vi "PC Vg Sweep.vi"() -> ()   [LabVIEW 2009]
uses:
  <vilib>/DAQmx/create/channels.llb/DAQmx Create Channel (AO-Voltage-Basic).vi
  <vilib>/DAQmx/create/channels.llb/DAQmx Create Channel (AI-Voltage-Basic).vi
  <vilib>/DAQmx/configure/timing.llb/DAQmx Timing (Sample Clock).vi
  <vilib>/DAQmx/write.llb/DAQmx Write (Analog DBL 1Chan 1Samp).vi
  <vilib>/DAQmx/read.llb/DAQmx Read (Analog 1D DBL 1Chan NSamp).vi
  <vilib>/Utility/file.llb/Write To Spreadsheet File (DBL).vi
  <vilib>/Analysis/NI_AALBase.lvlib
panel:
  in  "Stop":bool
  out "Vg":dbl(graph)
  out "Vsd":dbl(graph)
  out "Writing Vsd":bool
  out "Start Vsd Ramp":bool=TRUE
  in  "Measured Current":tag
  in  "Save Spectral?":bool
  in  "Save Map?":bool
  out "Mono Outputs":T1
  in  "Select Grating Blaze":string(combo)
  in  "Force\nInitialization (Def: F)":bool
  in  "Mono ID":string(combo)
  in  "Current Map":path
  in  "Spectral Response":path
  out "Current vs Wavelength":cluster{dbl[], dbl[]}(graph)
  out "Current vs Gate Voltage":cluster{dbl[], dbl[]}(graph)
  out "Out of Range":bool
  out "Vsd Ramp Position":cluster{"Vsd On":dbl, "Vsd On Vg Dir":bool}
  out "Recording":bool=TRUE
  out "Direction":bool=TRUE
  in  "Start Scan":bool
  out "Vsd Value (V)":dbl format="%0.2f"
  out "Vg Value (V)":dbl format="%0.2f"
  in  "Scan Values":T2={"Min Vg (V)"=0.0, "Max Vg (V)"=10.0, "Vm Start (V)"=5.0, "Vm Stop (V)"=9.0, "Steps/Sec"=100.0, "Vm Rate (Hz)"=100.0, "Wavelength Start (nm)"=450.0, "Wavelength Stop (nm)"=850.0, "Wavelength Step (nm)"=2.0, "Vsd (V)"=0.1, "Vg Step Size"=0.01, "Vsd Ramp Time (secs)"=0.1} {"Vsd Ramp Time (secs)" min=-10.0 max=10.0; "Vg Step Size" min=0.0 max=0.5; "Vsd (V)" min=-10.0 max=10.0; "Wavelength Step (nm)" min=0.0 max=500.0; "Wavelength Stop (nm)" min=16.0 max=2500.0; "Wavelength Start (nm)" min=15.0 max=2499.0; "Steps/Sec" min=1.0 max=1000.0; "Vm Stop (V)" min=-10.0 max=10.0; "Vm Start (V)" min=-10.0 max=10.0; "Max Vg (V)" min=-9.9 max=10.0; "Min Vg (V)" min=-10.0 max=9.9}
  in  "Start Mono":bool
  in  "Gate Voltage":tag
  in  "Source Drain Bias":tag
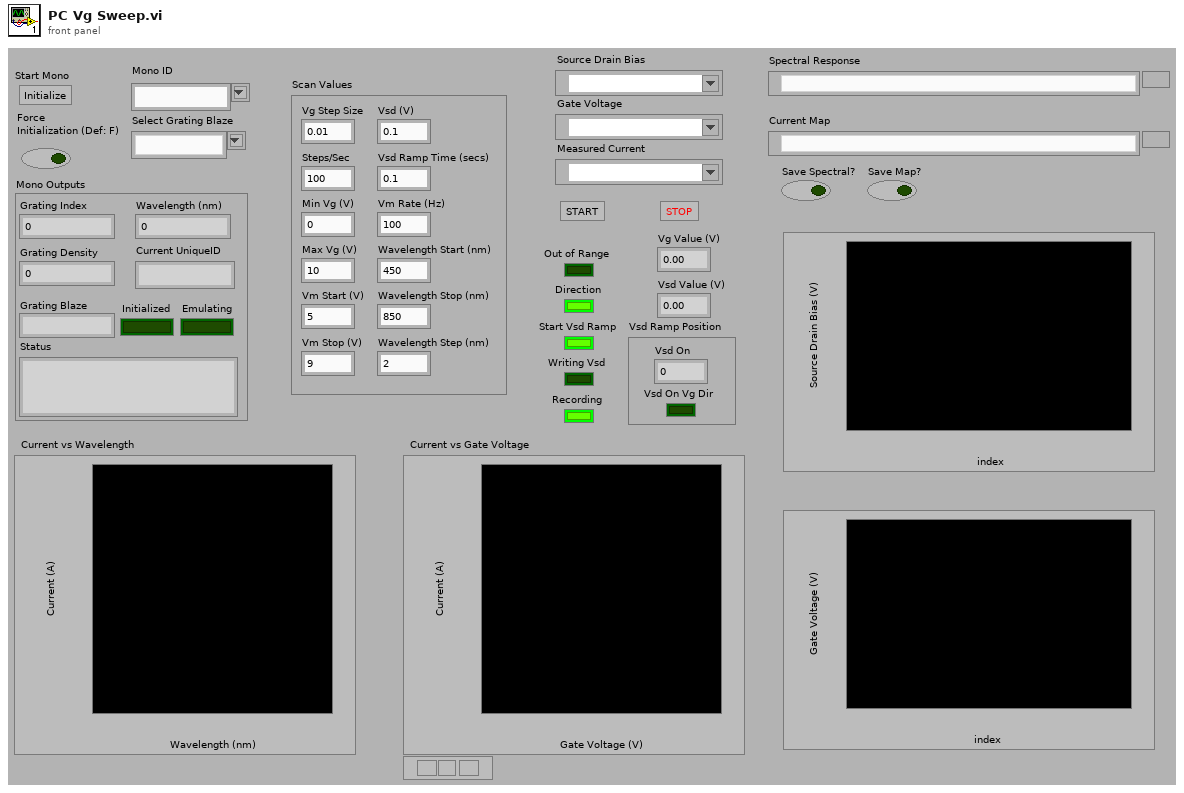
[diagram p1: front panel]
types:
  T1 = cluster{"Current UniqueID":string, "Current Blaze":string, "Grating Density":dbl, "Grating Index":i32, "Wavelength (nm)":dbl, "Emulating":bool, "Initialized":bool, "Status":string, "Refnum out":refnum<k7>}
  T2 = cluster{"Min Vg (V)":dbl, "Max Vg (V)":dbl, "Vm Start (V)":dbl, "Vm Stop (V)":dbl, "Steps/Sec":dbl, "Vm Rate (Hz)":dbl, "Wavelength Start (nm)":dbl, "Wavelength Stop (nm)":dbl, "Wavelength Step (nm)":dbl, "Vsd (V)":dbl, "Vg Step Size":dbl, "Vsd Ramp Time (secs)":dbl}
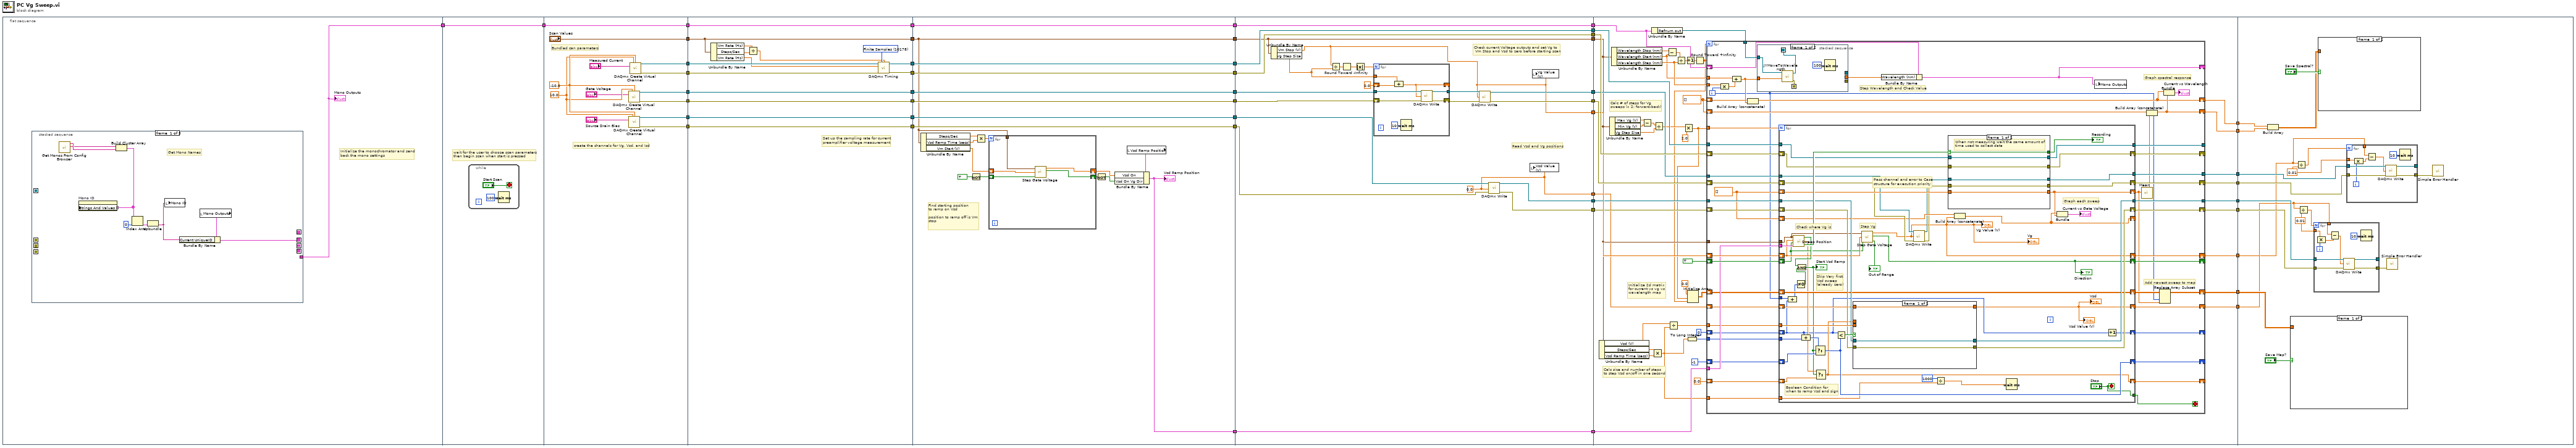
[diagram p0: block diagram]
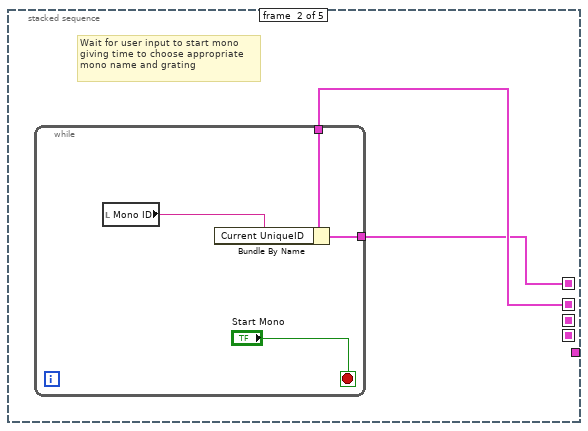
[diagram p2: hidden frame]
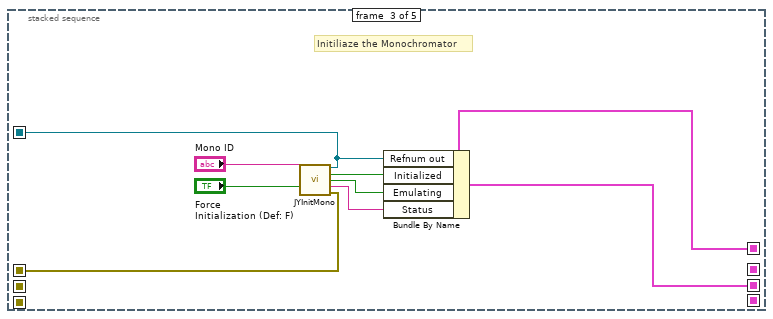
[diagram p3: hidden frame]
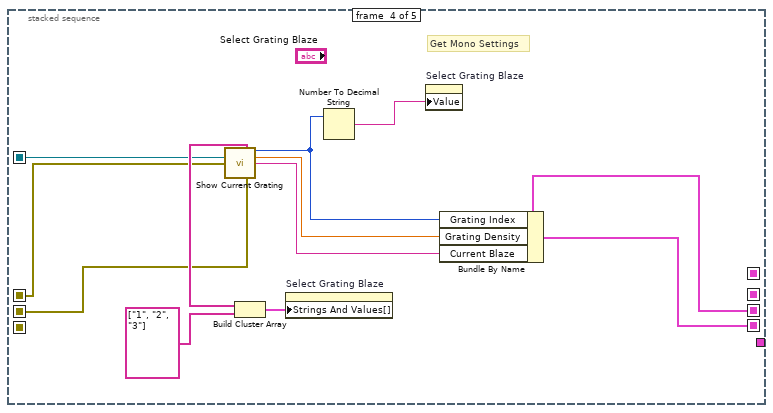
[diagram p4: hidden frame]
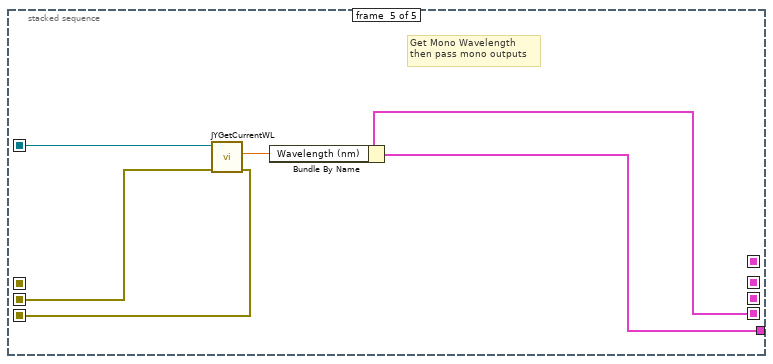
[diagram p5: hidden frame]
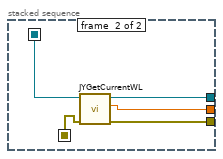
[diagram p6: hidden frame]
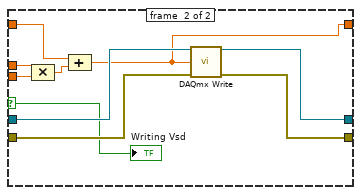
[diagram p7: hidden frame]
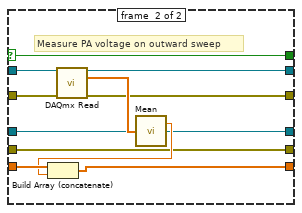
[diagram p8: hidden frame]
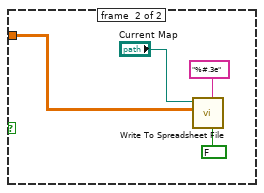
[diagram p9: hidden frame]
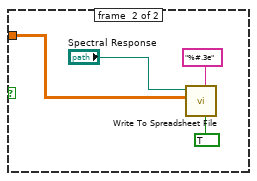
[diagram p10: hidden frame]
diagram:
  n1 = flat-sequence {
    tunnel: [w48] -> w2
    tunnel: w2 -> [w90]
    tunnel: [w90] -> w1
    tunnel: w1 -> [w101]
    tunnel: [w101] -> w47
    tunnel: ["Scan Values"] -> w46
    tunnel: [w99] -> w45
    tunnel: [w98] -> w44
    tunnel: [w97] -> w43
    tunnel: [w96] -> w42
    tunnel: [w95] -> w41
    tunnel: [w94] -> w40
    tunnel: [w120] -> w29
    tunnel: [w110] -> w27
    tunnel: [w119] -> w25
    tunnel: [w118] -> w23
    tunnel: [w117] -> w21
    tunnel: [w116] -> w19
    tunnel: [w114] -> w17
    tunnel: [w115] -> w15
    tunnel: w40 -> [w113]
    tunnel: w41 -> [w112]
    tunnel: w42 -> [w116]
    tunnel: w43 -> [w117]
    tunnel: w44 -> [w118]
    tunnel: w45 -> [w119]
    tunnel: w46 -> [w110]
    tunnel: w47 -> [w120]
    tunnel: w29 -> [w139]
    tunnel: [w139] -> w28
    tunnel: w27 -> [w132]
    tunnel: [w132] -> w26
    tunnel: w25 -> [w138]
    tunnel: [w138] -> w24
    tunnel: w23 -> [w137]
    tunnel: [w137] -> w22
    tunnel: w21 -> [w136]
    tunnel: [w136] -> w20
    tunnel: w19 -> [w135]
    tunnel: [w135] -> w18
    tunnel: w17 -> [w134]
    tunnel: [w134] -> w16
    tunnel: w15 -> [w133]
    tunnel: [w133] -> w14
    tunnel: [w125] -> w13
    tunnel: w28 -> [w164]
    tunnel: w26 -> [w158]
    tunnel: w24 -> [w149]
    tunnel: w22 -> [w153]
    tunnel: w20 -> [w148]
    tunnel: w18 -> [w152]
    tunnel: w16 -> [w162]
    tunnel: w14 -> [w163]
    tunnel: [w164] -> w39
    tunnel: [w145] -> w38
    tunnel: [w146] -> w37
    tunnel: [w155] -> w36
    tunnel: [w154] -> w35
    tunnel: [w163] -> w34
    tunnel: [w162] -> w33
    tunnel: [w150] -> w32
    tunnel: [w147] -> w31
    tunnel: [w158] -> w30
    tunnel: w13 -> [w156]
    tunnel: [w156] -> w12
    tunnel: w33 -> [w216]
    tunnel: w34 -> [w215]
    tunnel: w39 -> [w217]
    tunnel: w32 -> [w208]
    tunnel: w36 -> [w209]
    tunnel: w35 -> [w210]
    tunnel: w31 -> [w197]
    tunnel: w38 -> [w206]
    tunnel: w37 -> [w205]
    tunnel: w30 -> [w199]
    tunnel: w12 -> [w202]
    tunnel: [w189] -> w11
    tunnel: [w188] -> w10
    tunnel: [w187] -> w9
    tunnel: [w186] -> w8
    tunnel: [w185] -> w7
    tunnel: [w184] -> w6
    tunnel: [w183] -> w5
    tunnel: [w182] -> w4
    tunnel: [w181] -> w3
    tunnel: w11 -> [w380]
    tunnel: w10 -> [w379]
    tunnel: w9 -> [w377]
    tunnel: w8 -> [w370]
    tunnel: w7 -> [w369]
    tunnel: w6 -> [w368]
    tunnel: w5 -> [w367]
    tunnel: w4 -> [w366]
    tunnel: w3 -> [w365]
    frame #0 {
      # "Initialize the monochromator and send\nback the mono settings"
      n2 = stacked-sequence {
        seq-local: [_ _ w70 _ _] -> [_ _ _ w79 _]
        seq-local: [_ _ w69 _ _] -> [_ _ _ w78 w89]
        seq-local: [_ _ _ w77 _] -> [_ _ _ _ w88]
        seq-local: [_ _ _ _ w87] -> [_ _ _ _ _]
        seq-local: [w49 _ _ _ _] -> [_ w58 _ _ _]
        seq-local: [_ _ w64 _ _] -> [_ _ _ w76 _]
        seq-local: [_ _ _ w72 _] -> [_ _ _ _ w86]
        seq-local: [_ w57 _ _ _] -> [_ _ w63 _ _]
        tunnel: [_ _ _ _ w84] -> w48
        frame #0 {
          # "Get Mono Names"
          n3 = call "Get Monos From Config Browser.vi"() -> ("UniqueIDs"=w53:string[], "Mono ID"=w52:string[])  [unwired: 3 in, 1 out]
          n4 = Build Cluster Array(w52, w53) -> (w55:cluster{"String":string, "String":string}[])
          n5 = property on="Mono ID" class="CmbBox"("Strings And Values []"=w55) -> ()  [unwired: 2 in, 2 out]
          n6 = Index Array(array=w55, index=0) -> (element=w54:cluster{"String":string, "String":string})
          n7 = Unbundle(w54) -> ("String"=w50:string)  [unwired: 1 out]
          n8 = local write "Mono ID"(w50) -> ()
          n9 = local read "Mono Outputs"() -> (w51:T1)
          n10 = Bundle By Name(cluster=w51, "Current UniqueID"=w50) -> (w49:T1)
        }
        frame #1 {
          # "Wait for user input to start mono\ngiving time to choose appropriate\nmono name and grating"
          n11 = while {
            tunnel: w58 -> [w61]
            tunnel: [w59] -> w57
            stop <- "Start Mono" stop-if-true
            n12 = local read "Mono ID"() -> (w60:string)
            n13 = Bundle By Name(cluster=w61, "Current UniqueID"=w60) -> (w59:T1)
          }
        }
        frame #2 {
          # "Initiliaze the Monochromator"
          n14 = call "JYInitMono.vi"("Unique ID"="Mono ID", "Force Init"="Force\nInitialization (Def: F)") -> ("Mono RefNum out"=w69:refnum<k7>, "Initialized"=w68:bool, "Emulating"=w67:bool, "Status"=w66:string, "error out"=w70:errorcluster)  [unwired: 9 in]
          n15 = Bundle By Name(cluster=w63, "Refnum out"=w69, "Initialized"=w68, "Emulating"=w67, "Status"=w66) -> (w64:T1)
        }
        frame #3 {
          # "Get Mono Settings"
          n16 = call "Show Current Grating.vi"("Refnum in"=w78, "error in (no error)"=w79) -> ("Blazes"=w82:string[], "Grating Index"=w75:i32, "Current Grating"=w74:dbl, "Current Blaze"=w73:string, "error out"=w77:errorcluster)  [unwired: 5 in, 4 out]
          n17 = Build Cluster Array(w82, string[] ["1", "2", "3"]) -> (w80:cluster{"String":string, string}[])
          n18 = property on="Select Grating Blaze" class="CmbBox"("Strings And Values[]"=w80) -> ()  [unwired: 2 in, 2 out]
          n19 = Number To Decimal String(number=w75) -> (decimal integer string=w83:string)  [unwired: 1 in]
          n20 = property on="Select Grating Blaze" class="CmbBox"("Value"=w83) -> ()  [unwired: 2 in, 2 out]
          n21 = Bundle By Name(cluster=w76, "Grating Index"=w75, "Grating Density"=w74, "Current Blaze"=w73) -> (w72:T1)
        }
        frame #4 {
          # "Get Mono Wavelength\nthen pass mono outputs"
          n22 = call "JYGetCurrentWL.vi"("error in (no error)"=w88, "JYMONOLib.IJYMonoReqd"=w89) -> ("error out"=w87:errorcluster, "Current WL"=w85:dbl)  [unwired: 6 in, 2 out]
          n23 = Bundle By Name(cluster=w86, "Wavelength (nm)"=w85) -> (w84:T1)
        }
      }
      "Mono Outputs" <- w48
    }
    frame #1 {
      # "wait for the user to choose scan parameters\nthen begin scan when start is pressed"
      n24 = while {
        stop <- "Start Scan" stop-if-true
        n25 = Wait (ms)(milliseconds to wait=u32 100) -> ()  [unwired: 1 out]
      }
    }
    frame #2 {
      w105 = -10.0 ("maximum value")
      w104 = 10.0 ("maximum value")
      # "create the channels for Vg, Vsd, and Isd"
      # "Bundled can parameters"
      n26 = call-poly <vilib>:"DAQmx Create Virtual Channel.vi"("maximum value"=w104, "minimum value"=w105, "physical channels"="Gate Voltage") -> ("task out"=w98:refnum<k21>, "error out"=w96:errorcluster)  [unwired: 11 in]
      n27 = call-poly <vilib>:"DAQmx Create Virtual Channel.vi"("maximum value"=w104, "minimum value"=w105, "physical channels"="Source Drain Bias") -> ("task out"=w99:refnum<k21>, "error out"=w97:errorcluster)  [unwired: 11 in]
      n28 = call-poly <vilib>:"DAQmx Create Virtual Channel.vi"("maximum value"=w104, "minimum value"=w105, "physical channels"="Measured Current") -> ("task out"=w94:refnum<k21>, "error out"=w95:errorcluster)  [unwired: 11 in]
    }
    frame #3 {
      w111 = 10178 items=["Finite Samples"=10178, "Continuous Samples"=10123, "Hardware Timed Single Point"=12522] ("sample mode")
      # "Set up the sampling rate for current\npreamplifier voltage measurement"
      n29 = Unbundle By Name(w110) -> ("Vm Rate (Hz)"=w108:dbl, "Steps/Sec"=w109:dbl, "Vm Rate (Hz)"=w106:dbl)
      n30 = Divide(x=w108, y=w109) -> (x/y=w107:dbl)
      n31 = call-poly <vilib>:"DAQmx Timing.vi"("task/channels in"=w113, "sample mode"=w111, "samples per channel"=w107, "rate"=w106, "error in"=w112) -> ("task out"=w115:refnum<k21>, "error out"=w114:errorcluster)  [unwired: 9 in]
    }
    frame #4 {
      # "Find starting position\nto ramp on Vsd\n\nposition to ramp off is Vm\nstop"
      n32 = Unbundle By Name(w132) -> ("Steps/Sec"=w122:dbl, "Vsd Ramp Time (secs)"=w123:dbl, "Vm Start (V)"=w124:dbl)
      n33 = Not(x=TRUE ("Direction")) -> (.not. x?=w131:bool)
      n34 = Multiply(x=w122, y=w123) -> (x*y=w121:dbl)
      n35 = for {
        N: w121 -> [_]
        tunnel: w132 -> [w140]
        shift-right: [w143] -> w126
        shift-left: w124 -> [w144]
        shift-right: [w141] -> w129
        shift-left: w131 -> [w142]
        n36 = call "Step Gate Voltage.vi"("Scan Values"=w140, "Vg Value (V)"=w144, "Direction"=w142) -> ("New Vg Value (V)"=w143:dbl, "New Direction"=w141:bool)  [unwired: 2 out]
      }
      n37 = Not(x=w129) -> (.not. x?=w127:bool)
      n38 = local read "Vsd Ramp Position"() -> (w128:cluster{"Vsd On":dbl, "Vsd On Vg Dir":bool})
      n39 = Bundle By Name(cluster=w128, "Vsd On"=w126, "Vsd On Vg Dir"=w127) -> (w125:cluster{"Vsd On":dbl, "Vsd On Vg Dir":bool})
      "Vsd Ramp Position" <- w125
    }
    frame #5 {
      w147 = 0.0 ("data")
      # "Read Vsd and Vg positions"
      # "Check current Voltage outputs and set Vg to\n Vm Stop and Vsd to zero before starting scan"
      n40 = Unbundle By Name(w158) -> ("Vm Stop (V)"=w150:dbl, "Vg Step Size"=w157:dbl)
      n41 = Divide(x=w150, y=w157) -> (x/y=w161:dbl)
      n42 = Round Toward -Infinity(1:w161) -> (0:w160:dbl)
      n43 = Absolute Value(x=w160) -> (abs(x)=w159:dbl)
      n44 = for {
        N: w159 -> [_]
        tunnel: w153 -> [w174]
        tunnel: w157 -> [w167]
        tunnel: [w171] -> w166
        shift-right: [w170] -> w165
        shift-left: w152 -> [w173]
        shift-right: [w168] -> _
        shift-left: 0.0 -> [w169]
        n45 = Compound Arithmetic op=ADD(w167, w169) -> (w168:dbl)
        n46 = Wait (ms)(milliseconds to wait=u32 10) -> ()  [unwired: 1 out]
        n47 = call-poly <vilib>:"DAQmx Write.vi"("task/channels in"=w174, "data"=w168, "error in"=w173) -> ("task out"=w171:refnum<k21>, "error out"=w170:errorcluster)  [unwired: 10 in, 1 out]
      }
      n48 = call-poly <vilib>:"DAQmx Write.vi"("task/channels in"=w166, "data"=w150, "error in"=w165) -> ("task out"=w155:refnum<k21>, "error out"=w154:errorcluster)  [unwired: 10 in, 1 out]
      n49 = call-poly <vilib>:"DAQmx Write.vi"("task/channels in"=w149, "data"=w147, "error in"=w148) -> ("task out"=w145:refnum<k21>, "error out"=w146:errorcluster)  [unwired: 10 in, 1 out]
      n50 = local write "Vsd Value (V)"(w147) -> ()
      n51 = local write "Vg Value (V)"(w150) -> ()
    }
    frame #6 {
      w190 = dbl[] []
      # "Initialize 2d matrix\nfor current vs vg vs \nwavelength map"
      # "Calc # of steps for Vg\nsweeps (x 2: forward-back)"
      # "Calc size and number of steps\nto step Vsd on/off in one second"
      n52 = Unbundle By Name(w199) -> ("Vsd (V)"=w196:dbl, "Steps/Sec"=w177:dbl, "Vsd Ramp Time (secs)"=w176:dbl)
      n53 = Unbundle By Name(w199) -> ("Max Vg (V)"=w211:dbl, "Min Vg (V)"=w212:dbl, "Vg Step Size"=w213:dbl)
      n54 = Unbundle By Name(w199) -> ("Wavelength Stop (nm)"=w222:dbl, "Wavelength Start (nm)"=w219:dbl, "Wavelength Step (nm)"=w220:dbl)
      n55 = Subtract(x=w211, y=w212) -> (x-y=w214:dbl)
      n56 = Unbundle By Name(w217) -> ("Refnum out"=w218:refnum<k7>)
      n57 = Multiply(x=w177, y=w176) -> (x*y=w175:dbl)
      n58 = Divide(x=w214, y=w213) -> (x/y=w204:dbl)
      n59 = Subtract(x=w222, y=w219) -> (x-y=w221:dbl)
      n60 = Divide(x=w196, y=w175) -> (x/y=w195:dbl)
      n61 = Divide(x=w221, y=w220) -> (x/y=w201:dbl)
      n62 = Multiply(x=w204, y=2.0) -> (x*y=w192:dbl)
      n63 = Increment(x=w201) -> (x+1=w200:dbl)
      n64 = To Long Integer(number=w175) -> (32bit integer=w198:i32)
      n65 = Round Toward +Infinity(x=w200) -> (ceil(x): smallest int >= x=w193:dbl)
      n66 = Initialize Array(0.0, w192, w193) -> (w191:dbl[][])
      n67 = for {
        N: w193 -> [_]
        tunnel: w220 -> [w273]
        tunnel: w219 -> [w271]
        tunnel: w218 -> [w270]
        shift-right: [w233] -> _
        shift-left: w217 -> [w269]
        shift-right: [w238] -> w189
        shift-left: w190 -> [w244]
        shift-right: [w247] -> w183
        shift-left: w205 -> [w259]
        shift-right: [w246] -> w185
        shift-left: w210 -> [w266]
        tunnel: w206 -> [w260]
        tunnel: w209 -> [w267]
        tunnel: w215 -> [w256]
        shift-right: [w245] -> _
        shift-left: w216 -> [w255]
        tunnel: w198 -> [w254]
        tunnel: w192 -> [w265]
        shift-right: [w261] -> w181
        shift-left: w208 -> [w263]
        shift-right: [w262] -> _
        shift-left: TRUE -> [w264]
        tunnel: w202 -> [w258]
        tunnel: w199 -> [w257]
        shift-right: [w252] -> w182
        shift-left: w197 -> [w253]
        tunnel: w195 -> [w251]
        tunnel: [w250] -> w184
        tunnel: [w249] -> _
        tunnel: [w248] -> w186
        shift-right: [w235] -> w187
        shift-left: w191 -> [w243]
        shift-right: [w239] -> w188
        shift-left: w190 -> [w240]
        tunnel: w175 -> [w231]
        shift-right: [w226] -> _
        shift-left: 0 -> [w227]
        shift-right: [w224] -> _
        shift-left: -1 -> [w230]
        shift-right: [w225] -> _
        shift-left: 0.0 -> [w229]
        i -> [w228]
        stop <- w223 stop-if-true
        w242 = dbl[] []
        # "Add newest sweep to map"
        # "Step Wavelength and Check Value"
        # "Graph spectral response"
        n68 = Compound Arithmetic op=MULTIPLY(w273, w228) -> (w272:dbl)
        n69 = Compound Arithmetic op=ADD(w271, w272) -> (w268:dbl)
        n70 = Build Array (concatenate)(w244, w268) -> (w238:dbl[])
        n71 = stacked-sequence {
          seq-local: [w277 _] -> [_ w282]
          seq-local: [w276 _] -> [_ w283]
          tunnel: w270 -> [w278 _]
          tunnel: w268 -> [w275 _]
          tunnel: [_ w281] -> _
          tunnel: [_ w280] -> _
          tunnel: [_ w279] -> w232
          frame #0 {
            n72 = call "JYMoveToWavelength.vi"("Target WL"=w275, "RefNum In"=w278) -> ("error out"=w277:errorcluster, "Refnum Out"=w276:refnum<k7>)  [unwired: 2 in, 1 out]
            n73 = Wait (ms)(milliseconds to wait=u32 100) -> ()  [unwired: 1 out]
          }
          frame #1 {
            n74 = call "JYGetCurrentWL.vi"("error in (no error)"=w282, "JYMONOLib.IJYMonoReqd"=w283) -> ("error out"=w281:errorcluster, "Current WL"=w279:dbl, "Mono Refnum Out"=w280:refnum<k7>)  [unwired: 6 in, 1 out]
          }
        }
        n75 = for {
          N: w265 -> [_]
          tunnel: w267 -> [w313]
          shift-right: [w303] -> w246
          shift-left: w266 -> [w312]
          shift-right: [w290] -> w261
          shift-left: w263 -> [w317]
          shift-right: [w309] -> w262
          shift-left: w264 -> [w316]
          tunnel: w260 -> [w318]
          shift-right: [w310] -> w247
          shift-left: w259 -> [w319]
          tunnel: w258 -> [w334]
          tunnel: w257 -> [w284]
          tunnel: w256 -> [w331]
          shift-right: [w330] -> w245
          shift-left: w255 -> [w332]
          tunnel: [w329] -> w249
          shift-right: [w285] -> w234
          shift-left: w242 -> [w328]
          tunnel: w254 -> [w326]
          shift-right: [w324] -> w224
          shift-left: w230 -> [w325]
          shift-right: [w289] -> w252
          shift-left: w253 -> [w295]
          tunnel: w251 -> [w322]
          tunnel: [w311] -> w250
          tunnel: [w304] -> w248
          shift-right: [w286] -> _
          shift-left: w242 -> [w308]
          shift-right: [w307] -> w236
          shift-left: w243 -> [w307]
          tunnel: w231 -> [w301]
          shift-right: [w296] -> w225
          shift-left: w229 -> [w299]
          tunnel: w228 -> [w294]
          shift-right: [w292] -> w226
          shift-left: w227 -> [w291]
          tunnel: ["Stop"] -> w223
          stop <- "Stop" stop-if-true
          # "Boolean Condition for\nwhen to ramp Vsd and sign"
          # "Graph each sweep"
          # "Step Vg"
          # "Check where Vg is"
          # "Skip Very first\nVsd sweep \n(already zero)"
          # "Pass channel and error to Case\nstructure for execution priority"
          n76 = Compound Arithmetic op=ADD(w294, w291) -> (w293:i32)
          n77 = call "Sweep Position.vi"("Vsd Ramp Position"=w334, "Direction"=w316, "Vg Value (V)"=w317, "Scan Values"=w284) -> ("Recording"=w333:bool, "Vsd Ramp Sign"=w297:dbl, "Start Vsd Ramp"=w320:bool)
          n78 = Not Equal To 0?(x=w293) -> (x != 0?=w321:bool)
          n79 = And(x=w320, y=w321) -> (x .and. y?=w298:bool)
          "Start Vsd Ramp" <- w298
          n80 = Compound Arithmetic op=ADD(w291, w326) -> (w327:i32)
          n81 = Select(t=w327, s=w298, f=w325) -> (s? t:f=w324:i32)
          n82 = Select(t=w297, s=w298, f=w299) -> (s? t:f=w296:dbl)
          n83 = Less?(x=w291, y=w324) -> (x < y?=w323:bool)
          n84 = case shown="True" w323 {
            selector: w323 -> [_ w338]
            tunnel: w296 -> [_ w346]
            tunnel: w295 -> [w337 w344]
            tunnel: w322 -> [_ w347]
            tunnel: [w337 w341] -> w289
            tunnel: w319 -> [w335 w343]
            tunnel: w318 -> [w336 w342]
            tunnel: [w336 w339] -> w311
            tunnel: [w335 w340] -> w310
            frame #0 {
            }
            frame #1 {
              n85 = Compound Arithmetic op=MULTIPLY(w346, w347) -> (w345:dbl)
              n86 = Compound Arithmetic op=ADD(w344, w345) -> (w341:dbl)
              n87 = call-poly <vilib>:"DAQmx Write.vi"("task/channels in"=w342, "data"=w341, "error in"=w343) -> ("task out"=w339:refnum<k21>, "error out"=w340:errorcluster)  [unwired: 10 in, 1 out]
              "Writing Vsd" <- w338
            }
          }
          "Vsd Value (V)" <- w289
          "Vsd" <- w289
          n88 = call "Step Gate Voltage.vi"("Scan Values"=w284, "Vg Value (V)"=w317, "Direction"=w316) -> ("New Vg Value (V)"=w290:dbl, "New Direction"=w309:bool, "Out of Range"=→"Out of Range":bool)  [unwired: 1 out]
          "Vg Value (V)" <- w290
          "Direction" <- w309
          "Vg" <- w290
          n89 = call-poly <vilib>:"DAQmx Write.vi"("task/channels in"=w313, "data"=w290, "error in"=w312) -> ("task out"=w306:refnum<k21>, "error out"=w305:errorcluster)  [unwired: 10 in, 1 out]
          n90 = Divide(x=u32 1000 ("milliseconds to wait"), y=w301) -> (x/y=w300:dbl)
          n91 = case shown="True" w333 {
            selector: w333 -> [w350 w363]
            tunnel: w332 -> [w352 w357]
            tunnel: w331 -> [w353 w358]
            tunnel: [w353 w355] -> w329
            tunnel: [w352 w356] -> w330
            tunnel: w328 -> [w351 w364]
            tunnel: [w351 w354] -> w285
            tunnel: [w350 w363] -> w315
            tunnel: w306 -> [w349 w360]
            tunnel: w305 -> [w348 w359]
            tunnel: [w349 w360] -> w304
            tunnel: [w348 w359] -> w303
            frame #0 {
              # "When not measuring wait the same amount of \ntime used to collect data"
            }
            frame #1 {
              # "Measure PA voltage on outward sweep"
              n92 = call-poly <vilib>:"DAQmx Read.vi"("task/channels in"=w358, "error in"=w357) -> ("task out"=w355:refnum<k21>, "data"=w362:dbl[], "error out"=w356:errorcluster)  [unwired: 11 in]
              n93 = call <vilib>:"Mean.vi"("X"=w362) -> ("mean"=w361:dbl)  [unwired: 1 out]
              n94 = Build Array (concatenate)(w364, w361) -> (w354:dbl[])
            }
          }
          "Recording" <- w315
          n95 = Build Array (concatenate)(w308, w290) -> (w286:dbl[])
          n96 = Wait (ms)(milliseconds to wait=w300) -> ()  [unwired: 1 out]
          n97 = Bundle(w286, w285) -> (→"Current vs Gate Voltage":cluster{dbl[], dbl[]})  [unwired: 1 in]
          n98 = Increment(x=w291) -> (x+1=w292:i32)
        }
        n99 = Bundle By Name(cluster=w269, "Wavelength (nm)"=w232) -> (w233:T1)
        n100 = local write "Mono Outputs"(w233) -> ()
        n101 = call <vilib>:"Mean.vi"("X"=w234) -> ("mean"=w241:dbl)  [unwired: 1 out]
        n102 = Build Array (concatenate)(w240, w241) -> (w239:dbl[])
        n103 = Replace Array Subset(array=w236, new element=w234, index (col)=w228) -> (w235:dbl[][])  [unwired: 1 in]
        n104 = Bundle(w238, w239) -> (→"Current vs Wavelength":cluster{dbl[], dbl[]})  [unwired: 1 in]
      }
    }
    frame #7 {
      w373 = 0.01 ("y")
      w375 = 0.01 ("y")
      n105 = Build Array(w380, w379) -> (w378:dbl[][])
      n106 = case shown="True" "Save Map?" {
        tunnel: w377 -> [_ w403]
        frame #0 {
        }
        frame #1 {
          n107 = call-poly <vilib>:"Write To Spreadsheet File.vi"("transpose? (no:F)"=FALSE, "format (%.3f)"="%#.3e", "2D data"=w403, "file path (dialog if empty)"="Current Map") -> ()  [unwired: 4 in, 1 out]
        }
      }
      n108 = Divide(x=w365, y=w373) -> (x/y=w374:dbl)
      n109 = Divide(x=w366, y=w375) -> (x/y=w376:dbl)
      n110 = for {
        N: w376 -> [_]
        tunnel: w366 -> [w400]
        tunnel: w367 -> [w401]
        tunnel: w368 -> [w402]
        tunnel: w375 -> [w398]
        tunnel: [w395] -> w371
        tunnel: [w394] -> _
        i -> [w399]
        n111 = Compound Arithmetic op=MULTIPLY(w398, w399) -> (w397:dbl)
        n112 = Subtract(x=w400, y=w397) -> (x-y=w396:dbl)
        n113 = call-poly <vilib>:"DAQmx Write.vi"("task/channels in"=w402, "data"=w396, "error in"=w401) -> ("task out"=w394:refnum<k21>, "error out"=w395:errorcluster)  [unwired: 10 in, 1 out]
        n114 = Wait (ms)(milliseconds to wait=u32 10) -> ()  [unwired: 1 out]
      }
      n115 = case shown="True" "Save Spectral?" {
        tunnel: w378 -> [_ w407]
        frame #0 {
        }
        frame #1 {
          n116 = call-poly <vilib>:"Write To Spreadsheet File.vi"("transpose? (no:F)"=TRUE, "format (%.3f)"="%#.3e", "2D data"=w407, "file path (dialog if empty)"="Spectral Response") -> ()  [unwired: 4 in, 1 out]
        }
      }
      n117 = for {
        N: w374 -> [_]
        tunnel: w370 -> [w392]
        tunnel: w369 -> [w391]
        tunnel: [w390] -> w372
        tunnel: [w389] -> _
        tunnel: w373 -> [w387]
        tunnel: w365 -> [w385]
        i -> [w388]
        n118 = Compound Arithmetic op=MULTIPLY(w387, w388) -> (w386:dbl)
        n119 = Subtract(x=w385, y=w386) -> (x-y=w384:dbl)
        n120 = call-poly <vilib>:"DAQmx Write.vi"("task/channels in"=w392, "data"=w384, "error in"=w391) -> ("task out"=w389:refnum<k21>, "error out"=w390:errorcluster)  [unwired: 10 in, 1 out]
        n121 = Wait (ms)(milliseconds to wait=u32 10) -> ()  [unwired: 1 out]
      }
      n122 = call <vilib>:"Simple Error Handler.vi"("error in (no error)"=w371) -> ()  [unwired: 4 in, 5 out]
      n123 = call <vilib>:"Simple Error Handler.vi"("error in (no error)"=w372) -> ()  [unwired: 4 in, 5 out]
    }
  }
